vi "Initialize Attributes.vi"(8 "error in (no error)":errorcluster, 10 "Attribute Data":variant, 11 "CS++StartActor in":refnum<class "CS++StartActor.lvclass">) -> (0 "error out":errorcluster, 2 "Found?":bool, 3 "CS++StartActor out":refnum<class "CS++StartActor.lvclass">)   [LabVIEW 2012, in "CS++StartActor.lvlib" / "CS++StartActor.lvclass"]
doc: "Initialize object attribute.\n\nUnique resources should be allocated elsewhere!"
uses:
  CS++StartActor.lvclass
  CS++BaseActor/CS++BaseActor.lvclass
  CS++BaseActor/CS++BaseActor.lvclass/CS++BaseActor.ctl
  Classes/CS++BaseClasses/Factory/CS++Factory.lvclass
  CS++StartActor.lvclass/CS++StartActor.ctl
  Libraries/Base/CS++Base.lvlib
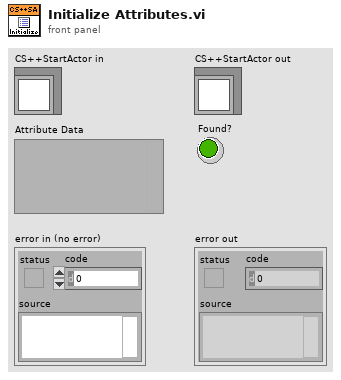
[diagram p1: front panel]
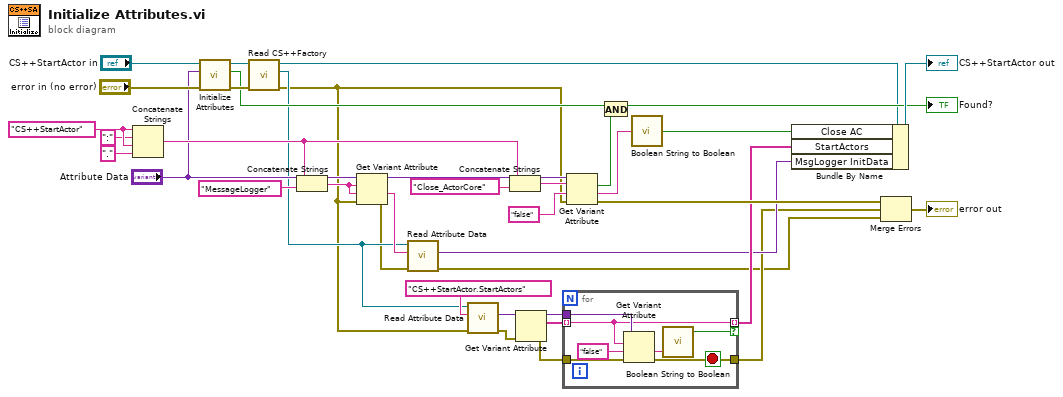
[diagram p0: block diagram]
diagram:
  w37 = "CS++StartActor"
  n1 = Concatenate Strings(w37, ":" ("string"), w37, "." ("string")) -> (w14:string)
  n2 = call-parent "Initialize Attributes.vi"("error in (no error)"="error in (no error)", "Attribute Data"="Attribute Data", "CS++BaseActor in"="CS++StartActor in") -> ("error out"=w8:errorcluster, "Found?"=w6:bool, "CS++BaseActor out"=w10:refnum<class "CS++StartActor.lvclass">)  [unwired: 6 in]
  n3 = call "Read CS++Factory.vi"("error in (no error)"=w8, "CS++BaseActor in"=w10) -> ("error out"=w3:errorcluster, "CS++Factory"=w5:refnum<class "CS++Factory.lvclass">, "CS++BaseActor out"=w9:refnum<class "CS++StartActor.lvclass">)  [unwired: 7 in]
  n4 = Concatenate Strings(w14, "MessageLogger" ("string")) -> (w15:string)
  n5 = Get Variant Attribute(Variant="Attribute Data", name=w15, default value (empty Variant)=w15, error in=w3) -> (duplicate Variant=w13:variant, value=w11:string, error out=w4:errorcluster)  [unwired: 1 out]
  n6 = call-dynamic "Read Attribute Data.vi"("error in (no error)"=w4, "Object Name"=w11, "CS++Factory in"=w5) -> ("error out"=w16:errorcluster, "Attribute Data"=w18:variant)  [unwired: 6 in, 1 out]
  n7 = call-dynamic "Read Attribute Data.vi"("error in (no error)"=w3, "Object Name"="CS++StartActor.StartActors" ("section"), "CS++Factory in"=w5) -> ("error out"=w23:errorcluster, "Attribute Data"=w24:variant)  [unwired: 6 in, 1 out]
  n8 = Concatenate Strings(w14, "Close_ActorCore" ("string")) -> (w34:string)
  n9 = Get Variant Attribute(Variant=w24, error in=w23) -> (duplicate Variant=w21:variant, names=w22:string[], error out=w20:errorcluster)  [unwired: 2 in, 1 out]
  n10 = for {
    tunnel: w22 -> [w44] mode=indexing
    tunnel: [w44] -> w19 mode=indexing if=w39
    tunnel: w21 -> [w45]
    tunnel: w20 -> [w43]
    tunnel: [w42] -> w17
    stop <- w42 stop-if-true
    n11 = Get Variant Attribute(Variant=w45, name=w44, default value (empty Variant)="false" ("string"), error in=w43) -> (value=w40:string, error out=w42:errorcluster)  [unwired: 2 out]
    n12 = call "Boolean String to Boolean.vi"("T/F String"=w40) -> ("Value"=w39:bool)
  }
  n13 = Get Variant Attribute(Variant=w13, name=w34, default value (empty Variant)="false" ("string"), error in=w3) -> (found=w29:bool, value=w2:string, error out=w28:errorcluster)  [unwired: 1 out]
  n14 = And(x=w6, y=w29) -> (x .and. y?=→"Found?":bool)
  n15 = call "Boolean String to Boolean.vi"("T/F String"=w2) -> ("Value"=w1:bool)
  n16 = Bundle By Name(cluster=w9, "Close AC"=w1, "StartActors"=w19, "MsgLogger InitData"=w18) -> (→"CS++StartActor out":refnum<class "CS++StartActor.lvclass">)
  n17 = Merge Errors(w28, w17, w16) -> (→"error out":errorcluster)
